vi "GAME START.vi"() -> (0 "stop 2":bool, 1 "User2 name 2":string, 3 "User1 name 2":string)   [LabVIEW 2014]
uses:
  gameover.ctl
panel:
  in  "User2 name":string
  in  "User1 name":string
  in  "stop":bool
  out "String":T1="GAME START"
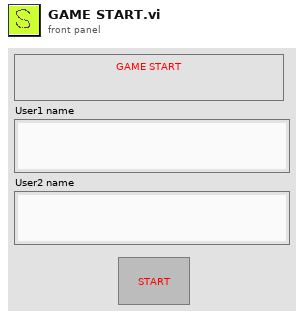
[diagram p1: front panel]
types:
  T1 = typedef "gameover.ctl" = string
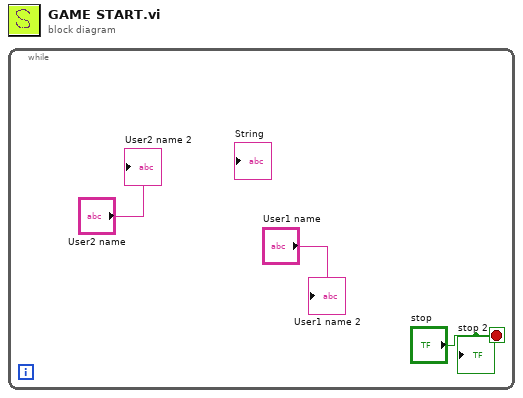
[diagram p0: block diagram]
diagram:
  n1 = while {
    stop <- "stop" stop-if-true
    "stop 2" <- "stop"
    "User2 name 2" <- "User2 name"
    "User1 name 2" <- "User1 name"
  }
